vi "Get Slaves.vi"(8 "error in (no error)":errorcluster, 11 "EtherCAT Master in":T3 {"VS ref" format="%.0x"}) -> (0 "error out":errorcluster, 1 "ECAT Generic Slaves":T2(array[cluster]) {"VS ref" format="%.0x"}, 2 "ECAT Slaves":T2(array[cluster]) {"VS ref" format="%.0x"}, 3 "EtherCAT Master out":T3 {"VS ref" format="%.0x"})   [LabVIEW 2016, in "Scan Engine Custom Device.lvlib"]
uses:
  Scan Engine Custom Device.lvlib
  <vilib>/NI Veristand/Custom Device API/Custom Device Item Ref.ctl
  Globals/Scan Engine GUIDs.vi
  <vilib>/NI Veristand/Custom Device API/Custom Device API.lvlib
  <resource>/objmgr/IndComECAT.rc
  <vilib>/NI Veristand/Custom Device Tools/Custom Device Utility Library/Custom Device Utility Library.lvlib
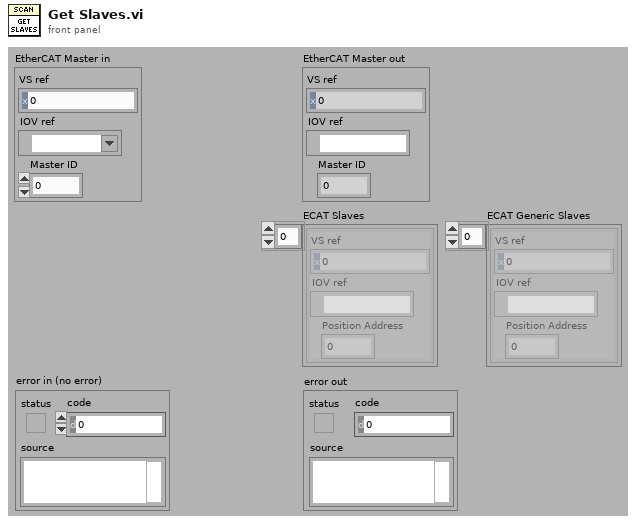
[diagram p1: front panel]
types:
  T1 = typedef "Custom Device API.lvlib/Custom Device Item Ref.ctl" = u64
  T2 = cluster{"VS ref":T1, "IOV ref":refnum<k21>, "Position Address":u16}[]
  T3 = cluster{"VS ref":T1, "IOV ref":refnum<k21>, "Master ID":u32}
  T4 = cluster{"ECAT Slave refs":T1[], "All ECAT Slaves":refnum<k21>[]}
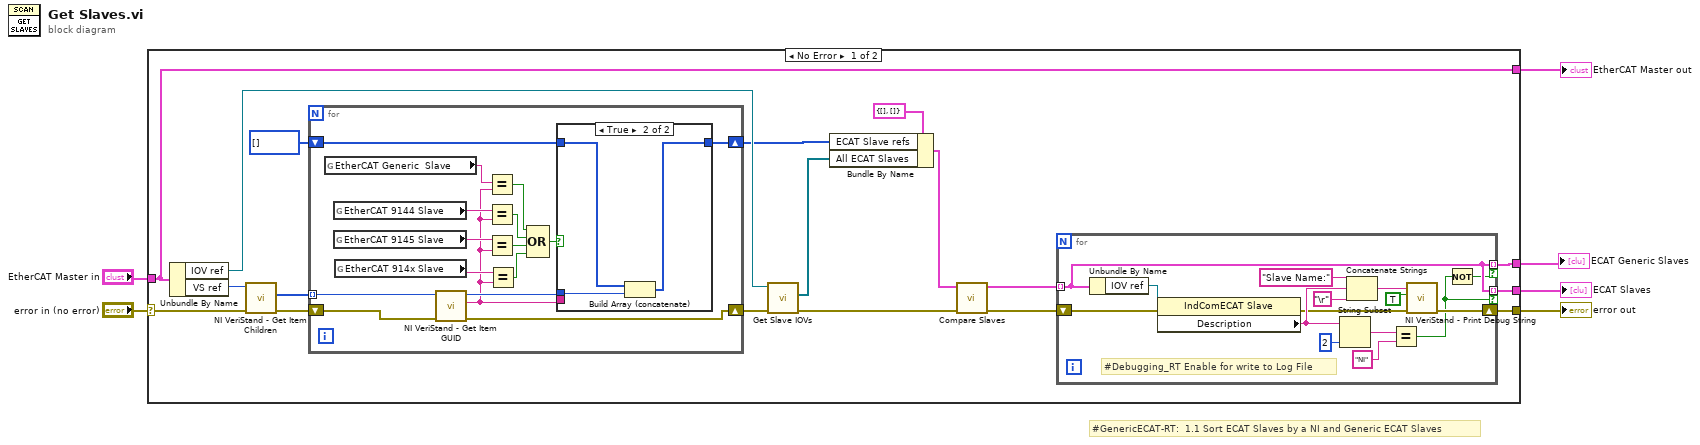
[diagram p0: block diagram]
diagram:
  # "#GenericECAT-RT:  1.1 Sort ECAT Slaves by a NI and Generic ECAT Slaves"
  n1 = case shown="No Error" "error in (no error)" {
    selector: "error in (no error)" -> [w21 w61]
    tunnel: [w8 w61] -> w6
    tunnel: [w14 w60] -> w3
    tunnel: "EtherCAT Master in" -> [w14 w60]
    tunnel: [w10 _] -> w2
    tunnel: [w9 _] -> w1
    frame No Error {
      n2 = Unbundle By Name(w14) -> ("IOV ref"=w16:refnum<k21>, "VS ref"=w17:T1)
      n3 = call <vilib>:"NI VeriStand - Get Item Children.vi"("error in (no error)"=w21, "Item Ref in"=w17) -> ("error out"=w22:errorcluster, "Child Refs"=w23:T1[])  [unwired: 6 in, 2 out]
      n4 = for {
        tunnel: w23 -> [w55] mode=indexing
        shift-right: [w51] -> w7
        shift-left: T1[] [] -> [w52]
        shift-right: [w49] -> w19
        shift-left: w22 -> [w50]
        n5 = global read "Scan Engine GUIDs.vi" "EtherCAT Generic  Slave"() -> (w46:string)
        n6 = global read "Scan Engine GUIDs.vi" "EtherCAT 9144 Slave"() -> (w41:string)
        n7 = global read "Scan Engine GUIDs.vi" "EtherCAT 9145 Slave"() -> (w42:string)
        n8 = global read "Scan Engine GUIDs.vi" "EtherCAT 914x Slave"() -> (w54:string)
        n9 = call <vilib>:"NI VeriStand - Get Item GUID.vi"("error in (no error)"=w50, "Item Ref in"=w55) -> ("error out"=w49:errorcluster, "GUID"=w40:string, "Item Ref out"=w53:T1)  [unwired: 7 in]
        n10 = Equal?(x=w46, y=w40) -> (x = y?=w45:bool)
        n11 = Equal?(x=w41, y=w40) -> (x = y?=w44:bool)
        n12 = Equal?(x=w42, y=w40) -> (x = y?=w43:bool)
        n13 = Equal?(x=w54, y=w40) -> (x = y?=w48:bool)
        n14 = Compound Arithmetic op=OR(w45, w44, w43, w48) -> (w47:bool)
        n15 = case shown="True" w47 {
          tunnel: w53 -> [_ w58]
          tunnel: w52 -> [w56 w59]
          tunnel: [w56 w57] -> w51
          tunnel: w40 -> [_ _]
          frame False {
          }
          frame True {
            n16 = Build Array (concatenate)(w59, w58) -> (w57:T1[])
          }
        }
      }
      n17 = call "Get Slave IOVs.vi"("error in (no error)"=w19, "ECAT Master in"=w16) -> ("error IO"=w13:errorcluster, "All Slaves"=w18:refnum<k21>[])  [unwired: 7 in, 1 out]
      n18 = Bundle By Name(cluster=T4 {"ECAT Slave refs"=[], "All ECAT Slaves"=[]} ("ECAT Slaves"), "ECAT Slave refs"=w7, "All ECAT Slaves"=w18) -> (w15:T4)
      n19 = call "Compare Slaves.vi"("error in (no error)"=w13, "ECAT Slaves in"=w15) -> ("error out"=w11:errorcluster, "ECAT Slaves out"=w12:T2)  [unwired: 8 in]
      n20 = for {
        tunnel: w12 -> [w34] mode=indexing
        tunnel: [w34] -> w9 mode=indexing if=w27
        tunnel: [w34] -> w10 mode=indexing if=w26
        shift-right: [w29] -> w8
        shift-left: w11 -> [w38]
        # "#Debugging_RT Enable for write to Log File"
        n21 = Unbundle By Name(w34) -> ("IOV ref"=w39:refnum<k21>)
        n22 = property class="IndComECAT Slave"(reference=w39, error in=w38) -> (error out=w25:errorcluster, "Description"=w31:string)  [unwired: 1 out]
        n23 = String Subset(string=w31, length (rest)=2 ("Länge (Rest)")) -> (substring=w36:string)  [unwired: 1 in]
        n24 = Concatenate Strings("Slave Name:", w31, "\r") -> (w30:string)
        n25 = Equal?(x=w36, y="NI" ("Nach String/Zeichen suchen (-)")) -> (x = y?=w26:bool)
        n26 = call <vilib>:"NI VeriStand - Print Debug String.vi"("error in (no error)"=w25, "Add to log file? (T)"=TRUE, "Message"=w30) -> ("error out"=w29:errorcluster)  [unwired: 8 in]
        n27 = Not(x=w26) -> (.not. x?=w27:bool)
      }
    }
    frame Error {
    }
  }
  "error out" <- w6
  "EtherCAT Master out" <- w3
  "ECAT Slaves" <- w2
  "ECAT Generic Slaves" <- w1
